vi "CreateSubpanelReference.vi"(8 "error in (no error)":errorcluster, 11 "EmbeddedMainUI in":refnum<class "EmbeddedMainUI.lvclass">) -> (0 "error out":errorcluster, 3 "EmbeddedMainUI out":refnum<class "EmbeddedMainUI.lvclass">)   [LabVIEW 2016, in "EmbeddedMainUI.lvclass"]
uses:
  EmbeddedMainUI.lvclass
  EmbeddedMainUI.lvclass/EmbeddedMainUI.ctl
  <vilib>/Levylab/Embedded SMO UI/EmbeddedSMO.lvclass
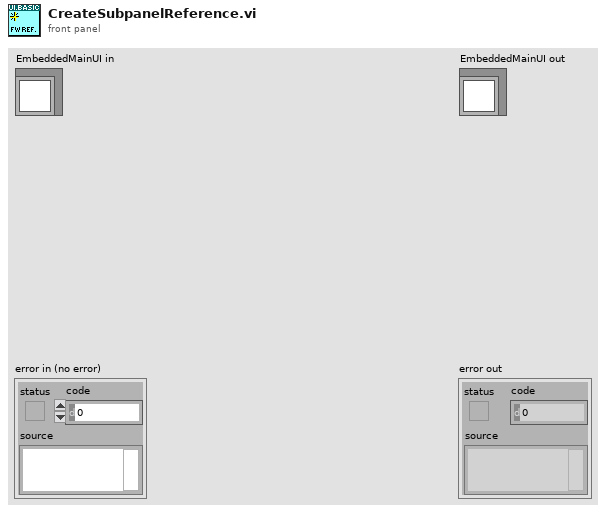
[diagram p1: front panel]
types:
  T1 = typedef "EmbeddedMainUI.lvclass/FrameworkDataRef.ctl" = refnum<data-value>
  T2 = typedef "EmbeddedMainUI.lvclass/FrameworkData.ctl" = cluster{"Subpanels":refnum<class "EmbeddedSMO.lvclass">[], "Left Subpanel":refnum<vi>, "Right Subpanel":refnum<vi>, "Active Left":i32, "Active Right":i32}
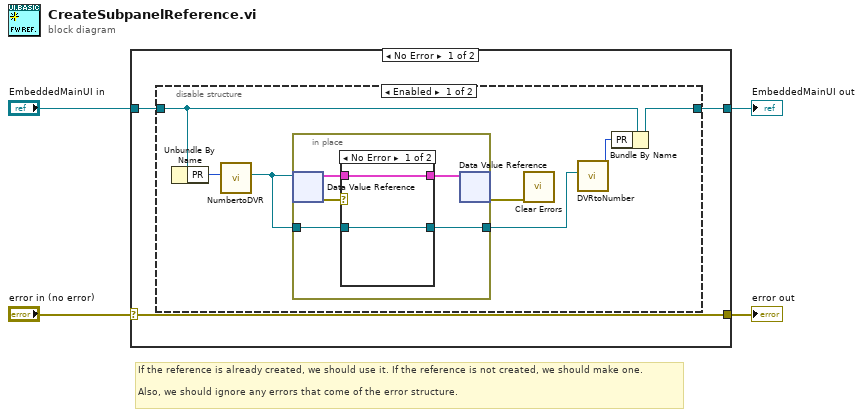
[diagram p0: block diagram]
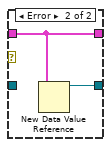
[diagram p2: hidden frame]
diagram:
  # "If the reference is already created, we should use it. If the reference is not created, we should make one. \n\nAlso, we should ignore any errors that come of the error structure."
  n1 = case shown="No Error" "error in (no error)" {
    selector: "error in (no error)" -> [w5 w26]
    tunnel: [w5 w26] -> w3
    tunnel: [w7 w25] -> w1
    tunnel: "EmbeddedMainUI in" -> [w6 w25]
    frame No Error {
      n2 = disable-structure shown="Enabled" {
        disable-tunnel: [w14 w24] -> w7
        disable-tunnel: w6 -> [w13 w24]
        frame Enabled {
          n3 = Unbundle By Name(w13) -> ("PR"=w9:i32)
          n4 = call "NumbertoDVR.vi"("Numeric"=w9) -> ("FrameworkDataRef"=w8:T1)  [unwired: 10 in]
          n5 = in-place {
            in-place-border: [w16] -> w10
            in-place-border: w8 -> [w15]
            n6 = in-place-dvr #1(w8) -> (w17:T2, w19:errorcluster)
            n7 = case shown="No Error" w19 {
              tunnel: [w21 w23] -> w18
              tunnel: w17 -> [w21 w23]
              tunnel: [w20 w22] -> w16
              tunnel: w15 -> [w20 _]
              frame No Error {
              }
              frame Error {
                n8 = New Data Value Reference(data value=w23) -> (data value reference=w22:refnum<data-value>)  [unwired: 1 in, 1 out]
              }
            }
            n9 = in-place-dvr #1(w18) -> (w12:errorcluster)  [unwired: 1 out]
          }
          n10 = call <vilib>:"Clear Errors.vi"("error in (no error)"=w12) -> ()  [unwired: 5 in, 2 out]
          n11 = call "DVRtoNumber.vi"("FrameworkDataRef"=w10) -> ("Number"=w11:i32)  [unwired: 10 in]
          n12 = Bundle By Name(cluster=w13, "PR"=w11) -> (w14:refnum<class "EmbeddedMainUI.lvclass">)
        }
        frame Disabled {
        }
      }
    }
    frame Error {
    }
  }
  "error out" <- w3
  "EmbeddedMainUI out" <- w1
